vi "ke37xx Revision Query.vi"(8 "error in (no error)":errorcluster, 11 "VISA resource name":refnum<visa-resource-name>) -> (0 "error out":errorcluster, 1 "Instr Firmware Revision":string, 2 "Instr Driver Revision":string, 3 "VISA resource name out":refnum<visa-resource-name>)   [LabVIEW 2009, in "Keithley 3700 Series.lvlib"]
doc: "This VI queries the current instrument firmware revision and instrument driver revision for the:\n\nKeithley 27xx Multimeter / Switch Unit (Integra Series)"
uses:
  <instrlib>/Keithley 3706/Keithley 3700 Series.lvlib
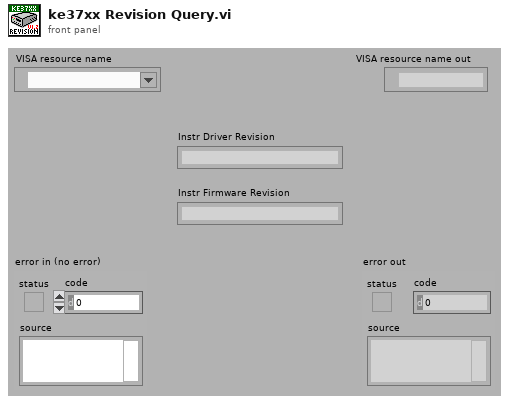
[diagram p1: front panel]
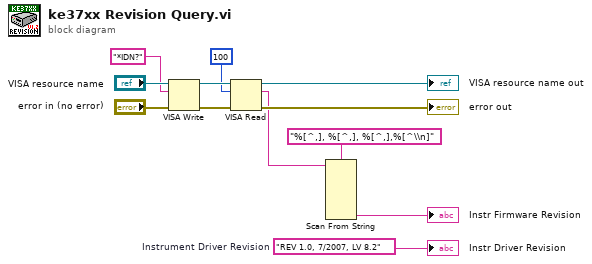
[diagram p0: block diagram]
diagram:
  w12 = "REV 1.0, 7/2007, LV 8.2"  # Instrument Driver Revision
  n1 = VISA Write(VISA resource name="VISA resource name", write buffer="*IDN?" ("Revision Query Command"), error in (no error)="error in (no error)") -> (VISA resource name out=w3:refnum<visa-resource-name>, error out=w4:errorcluster)  [unwired: 1 out]
  n2 = VISA Read(VISA resource name=w3, byte count=u32 100 ("Num Bytes to Read"), error in (no error)=w4) -> (VISA resource name out=→"VISA resource name out":refnum<visa-resource-name>, read buffer=w6:string, error out=→"error out":errorcluster)  [unwired: 1 out]
  n3 = Scan From String(format string="%[^,], %[^,], %[^,],%[^\\n]", input string=w6) -> (output 4=→"Instr Firmware Revision":string)  [unwired: 2 in, 10 out]
  "Instr Driver Revision" <- w12
